vi "Send Create Reference Message and Wait On Return.vi"(6 "timeout in ms (-1)":i32=-1, 8 "error in (no error)":errorcluster, 10 "Object":refnum<class>, 11 "Message Enqueuer in":refnum<class "Message Enqueuer.lvclass">) -> (0 "error out":errorcluster, 3 "Object Reference":refnum<data-value>)   [LabVIEW 2020, in "Create Ref Message.lvclass"]
uses:
  <vilib>/gpm_packages/@cs/Network-interface/Source/Create Ref Message/Create Ref Message.lvclass
  <vilib>/ActorFramework/Message Enqueuer/Message Enqueuer.lvclass
  C:/Program Files/National Instruments/LabVIEW 2020/vi.lib/ActorFramework/Message/Message.lvclass
  <vilib>/gpm_packages/@cs/Network-interface/Source/Create Ref Message/Create Ref Message.lvclass/Create Ref Message.ctl
  <vilib>/ActorFramework/Message Enqueuer/Message Enqueuer.lvclass/Message Enqueuer.ctl
  <vilib>/ActorFramework/Message Priority Queue/Priority Enqueue.vi
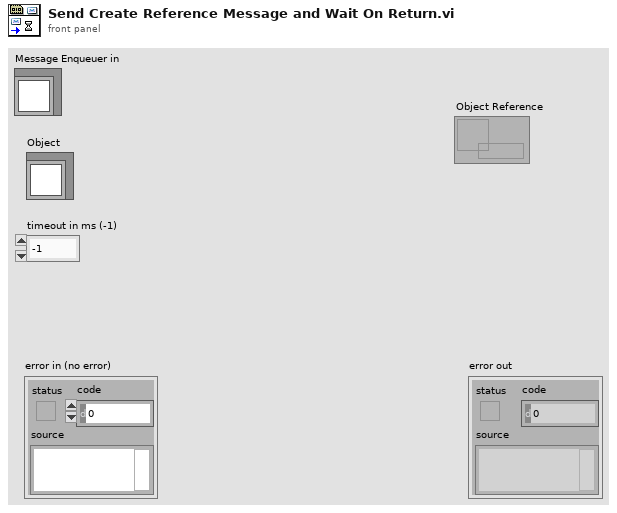
[diagram p1: front panel]
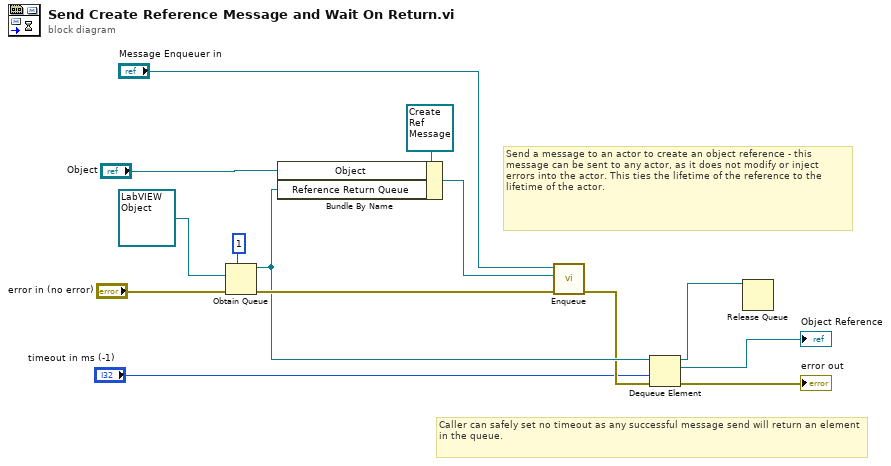
[diagram p0: block diagram]
diagram:
  # "Caller can safely set no timeout as any successful message send will return an element in the queue."
  # "Send a message to an actor to create an object reference - this message can be sent to any actor, as it does not modify or inject errors into the actor. This ties the lifetime of the reference to the lifetime of the actor."
  n1 = Obtain Queue(max queue size (-1, unlimited)=1, element data type=refnum<data-value> refnum ("data value reference"), error in (no error)="error in (no error)") -> (queue out=w7:refnum<queue>, error out=w9:errorcluster)  [unwired: 2 in, 1 out]
  n2 = Bundle By Name(cluster=refnum<class "Create Ref Message.lvclass"> refnum ("Create Ref Message in"), "Object"="Object", "Reference Return Queue"=w7) -> (w13:refnum<class "Create Ref Message.lvclass">)
  n3 = call <vilib>:"Enqueue.vi"("error in (no error)"=w9, "Message"=w13, "Message Enqueuer in"="Message Enqueuer in") -> ("error out"=w6:errorcluster)  [unwired: 7 in, 1 out]
  n4 = Dequeue Element(queue=w7, timeout in ms (-1)="timeout in ms (-1)", error in (no error)=w6) -> (queue out=w4:refnum<queue>, element=→"Object Reference":refnum<data-value>, error out=→"error out":errorcluster)  [unwired: 1 out]
  n5 = Release Queue(queue=w4) -> ()  [unwired: 2 in, 3 out]
